vi "remove channel from active array.vi"(2 "line to remove":u32, 3 "line array in":u32[](array[numeric])) -> (0 "removal":bool, 1 "line array out":u32[](array[numeric]))   [LabVIEW 2015]
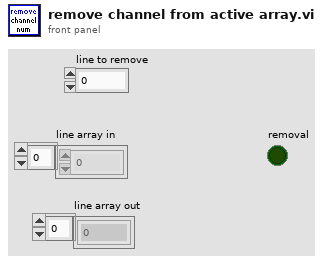
[diagram p1: front panel]
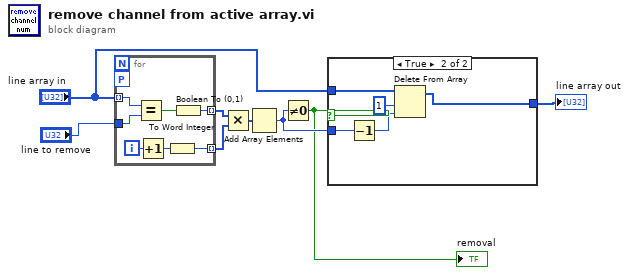
[diagram p0: block diagram]
diagram:
  n1 = for {
    workers-P: _ -> [_]
    tunnel: "line array in" -> [w14] mode=indexing
    tunnel: "line to remove" -> [w15]
    tunnel: [w10] -> w4 mode=indexing
    tunnel: [w11] -> w5 mode=indexing
    i -> [w13]
    n2 = Equal?(x=w14, y=w15) -> (x = y?=w12:bool)
    n3 = Increment(x=w13) -> (x+1=w9:i32)
    n4 = To Word Integer(number=w9) -> (16bit integer=w10:i16)
    n5 = Boolean To (0,1)(Boolean=w12) -> (0, 1=w11:i16)
  }
  n6 = Multiply(x=w5, y=w4) -> (x*y=w3:i16[])
  n7 = Add Array Elements(numeric array=w3) -> (sum=w2:i16)
  n8 = Not Equal To 0?(x=w2) -> (x != 0?=w1:bool)
  "removal" <- w1
  n9 = case shown="True" w1 {
    tunnel: "line array in" -> [w16 w21]
    tunnel: [w16 w18] -> w6
    tunnel: w2 -> [_ w20]
    frame False {
    }
    frame True {
      n10 = Decrement(x=w20) -> (x-1=w17:i16)
      n11 = Delete From Array(array=w21, length=1, index=w17) -> (array with subset deleted=w18:u32[])  [unwired: 1 out]
    }
  }
  "line array out" <- w6
